vi "Na-DAS_7609.vi"(3 "Timeout (ms)":u32=10000, 5 "Input voltage range (V)":u8(ring)=1 items=["-5... +5 V", "-10... +10 V"]) -> (0 "DAQ Error":errorcluster, 1 "Overruns":u32, 2 "Config read-back ok":bool)   [LabVIEW 2014]
doc: "Use this plug-in with the Nathan 7609 data acquisition system"
uses:
  Globals/Meas_global.vi
  PWA/PWAtasksGLOBAL.vi
  Globals/Trav_pos_global.vi
  Globals/Extra_Commands_Global.vi
  Globals/Dynamic_call_global.ph.vi
panel:
  # "PN 25/11/2014, 19/12/2014"
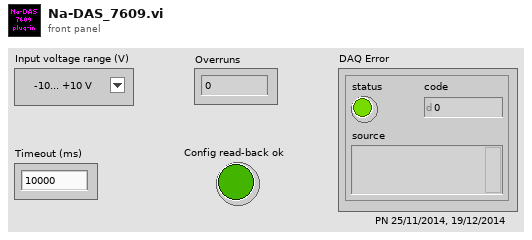
[diagram p1: front panel]
types:
  T1 = typedef "LDA_Setup.ctl" = cluster{"dimensions":enum16{"1D", "2D"}, "Analogue Freq Multiplier":dbl}
  T2 = typedef "Trigger_Mode.ctl" = enum16{"Free Running", "Start on Trigger", "Trigger Every Block", "Trigger Every Sample"}
  T3 = typedef "Traverse_cluster.ctl" = cluster{"Start X":dbl, "Start Y":dbl, "Start Z":dbl, "End X":dbl, "End Y":dbl, "End Z":dbl, "No. of pts.":i32, "Spacing":T4, "Filename":path, "Tunnel Speed":dbl, "Averaging time (min)":dbl, "Extra Commands":string, "Specific Arguments":string, "Emission Rate (l/min)":dbl, "Trace Gas Concentration (%)":dbl, "Density Ratio":string, "Comments":string, "Row No":i32, "Row Type Selector":T5, "Completion time":string, "Row Duration (mins)":dbl, "No. of Valid pts.":i32, "Meas Setup File":string}
  T4 = typedef "Spacing.ctl" = enum16{"Linear", "Log", "Gauss", "Specified", "N/A"}
  T5 = typedef "Multi_run_mode.ctl" = enum16{"Move Traverse Only", "Set Tunnel Speed Only", "Set Source Only", "Set Measurement Conditions", "Single Measurement", "Vertical Profile", "Lateral Profile", "Longitudinal Profile", "Explore Volume", "Multi-Axis Profile", "Auto Calibrate", "Meas Fast FID Bkgnd", "Check Beam Power", "Scanning Valve Measurement", "Run VI Named:", "Set ADAM Ch", "Wait (minutes)", "Send Message", "Synchronize With:", "Fall Back to this Row", "Turn Off Row Repeating", "Blank Row", "Traverse 3D Volume"}
  T6 = typedef "Ch_and_Spans.ctl" = cluster{"high limit (10V)":sgl, "low limit (-10V)":sgl, "Ch No":i16, "Var name":string, "Use Latest Calib":bool}
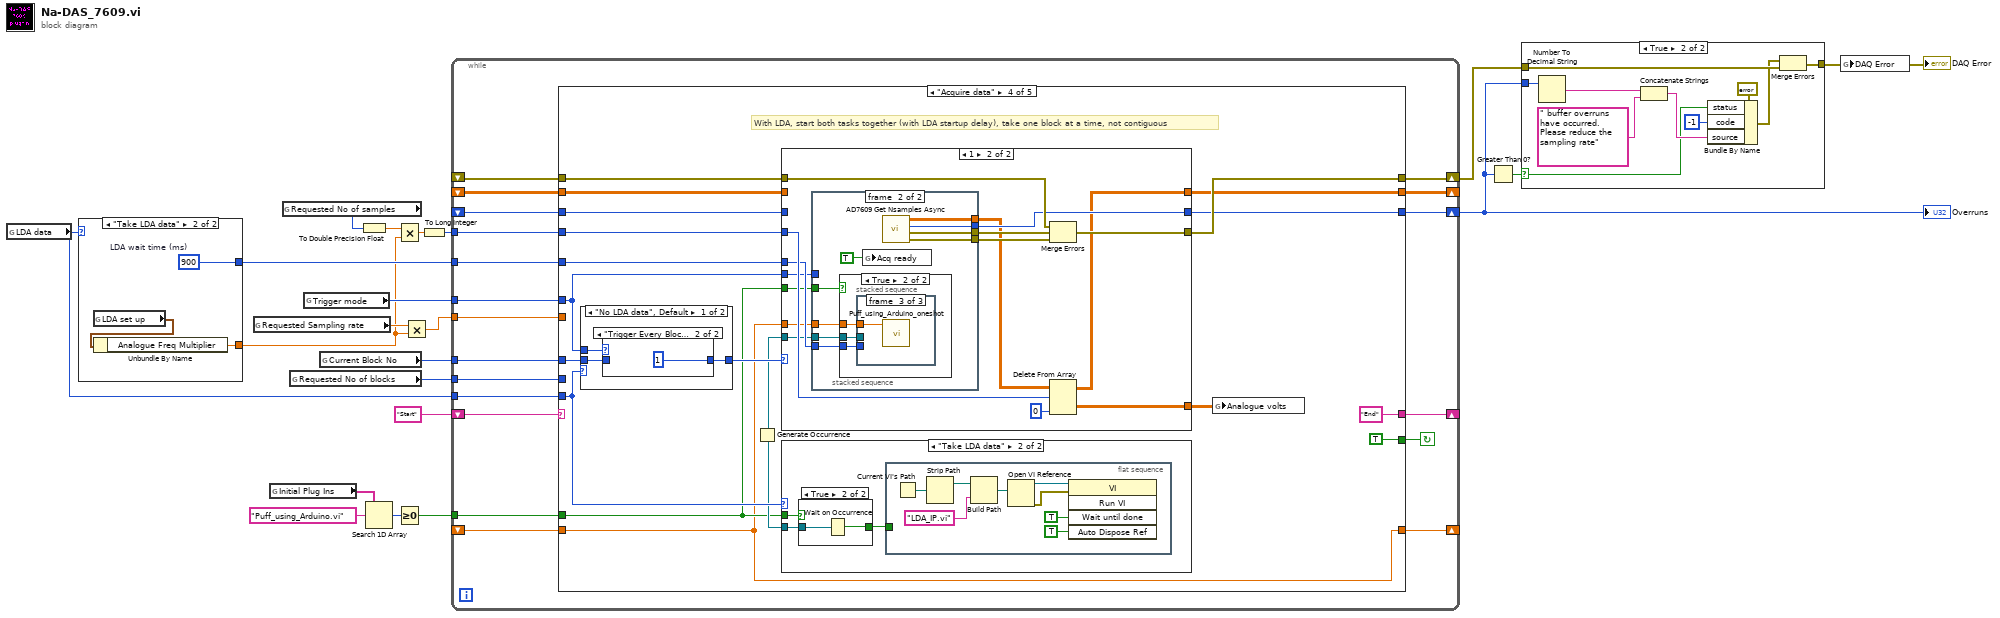
[diagram p0: block diagram]
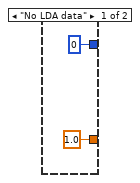
[diagram p3: hidden frame]
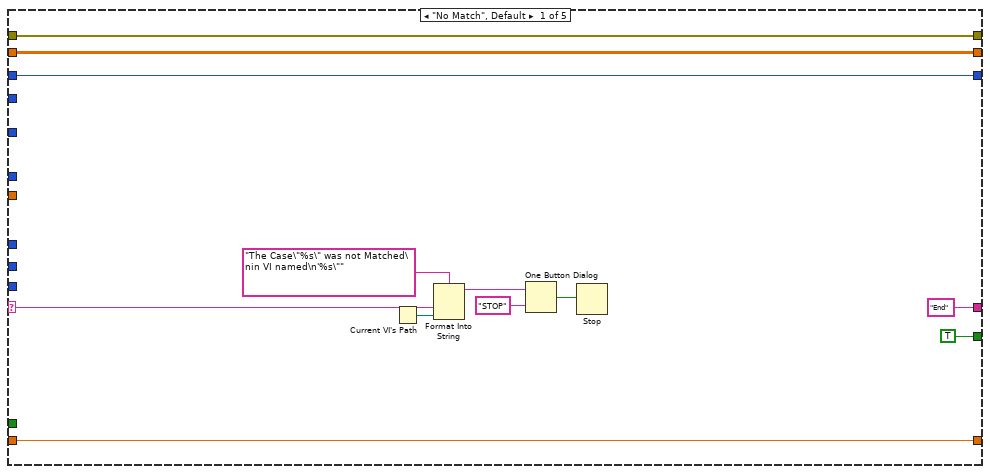
[diagram p4: hidden frame]
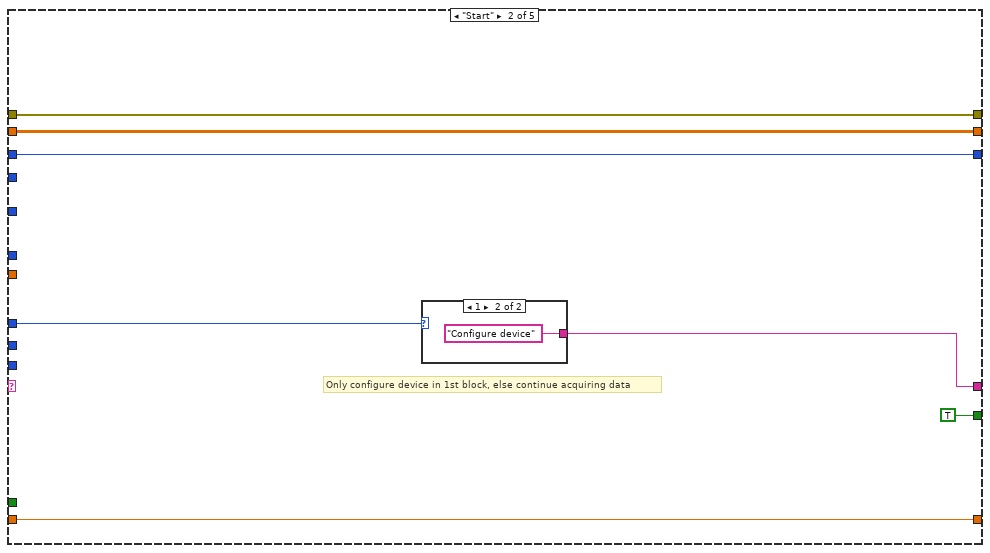
[diagram p5: hidden frame]
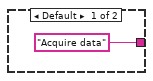
[diagram p6: hidden frame]
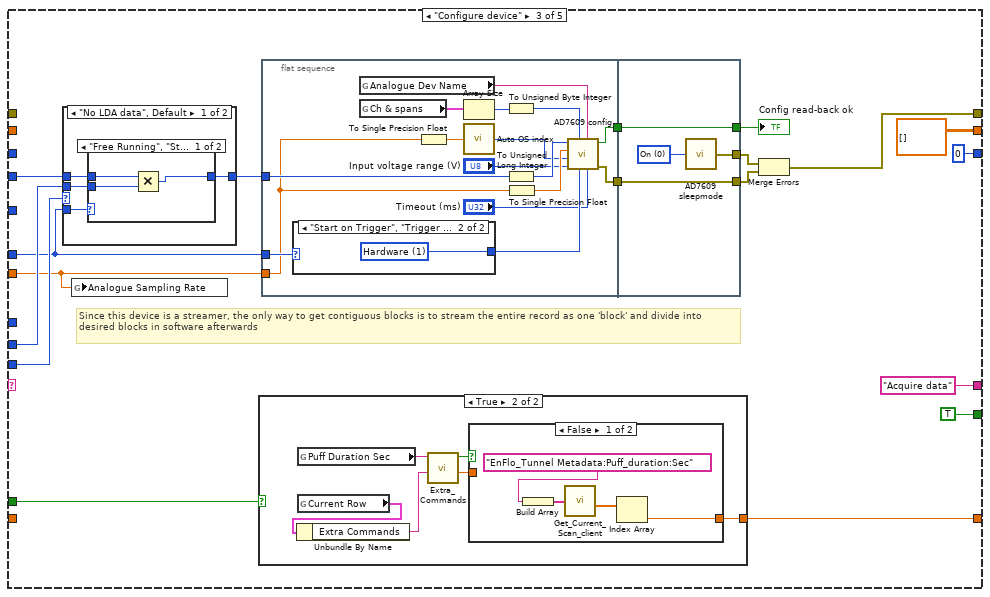
[diagram p7: hidden frame]
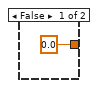
[diagram p8: hidden frame]
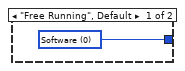
[diagram p12: hidden frame]
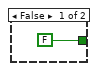
[diagram p14: hidden frame]
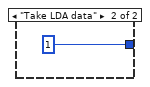
[diagram p16: hidden frame]
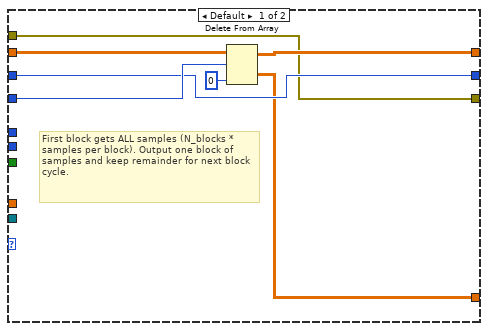
[diagram p17: hidden frame]
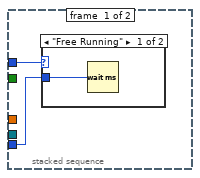
[diagram p18: hidden frame]
diagram:
  n1 = global read "Meas_global.vi" "LDA data"() -> (w16:enum16{"No LDA data", "Take LDA data"})
  n2 = case shown="\"Take LDA data\"" w16 {
    tunnel: [1.0 ("Analogue Freq Multiplier") w25] -> w5
    tunnel: [u32 0 ("LDA wait time (ms)") w24] -> w11
    frame "No LDA data" {
    }
    frame "Take LDA data" {
      w24 = u32 900  # LDA wait time (ms)
      n3 = global read "Meas_global.vi" "LDA set up"() -> (w26:T1)
      n4 = Unbundle By Name(w26) -> ("Analogue Freq Multiplier"=w25:dbl)
    }
  }
  n5 = global read "Meas_global.vi" "Requested Sampling rate"() -> (w17:dbl)
  n6 = global read "Dynamic_call_global.ph.vi" "Initial Plug Ins"() -> (w13:string[])
  n7 = global read "Meas_global.vi" "Requested No of samples"() -> (w6:i32)
  n8 = global read "Meas_global.vi" "Requested No of blocks"() -> (w1:i32)
  n9 = global read "Meas_global.vi" "Trigger mode"() -> (w20:T2)
  n10 = global read "Meas_global.vi" "Current Block No"() -> (w19:i32)
  n11 = To Double Precision Float(number=w6) -> (double precision float=w4:dbl)
  n12 = Search 1D Array(1D array=w13, element="Puff_using_Arduino.vi") -> (index of element=w15:i32)  [unwired: 1 in]
  n13 = Multiply(x=w4, y=w5) -> (x*y=w3:dbl)
  n14 = Greater Or Equal To 0?(x=w15) -> (x >= 0?=w12:bool)
  n15 = Multiply(x=w17, y=w5) -> (x*y=w18:dbl)
  n16 = To Long Integer(number=w3) -> (32bit integer=w2:i32)
  n17 = while {
    shift-left: "Start" -> [w45]
    shift-right: [w31] -> _
    tunnel: w18 -> [w44]
    tunnel: w2 -> [w43]
    tunnel: w19 -> [w42]
    tunnel: w20 -> [w40]
    tunnel: w16 -> [w39]
    tunnel: w1 -> [w38]
    shift-right: [w36] -> w10
    shift-left: _ -> [w37]
    shift-right: [w35] -> _
    shift-left: _ -> [w34]
    shift-right: [w33] -> w8
    shift-left: _ -> [w32]
    tunnel: w11 -> [w30]
    tunnel: w12 -> [w29]
    shift-right: [w28] -> _
    shift-left: _ -> [w27]
    stop <- w41 continue-if-true
    n18 = case shown="\"Acquire data\"" w45 {
      selector: w45 -> [w50 _ _ _ _]
      tunnel: ["End" w61 "Acquire data" ("f") "End" "End" ("f")] -> w31
      tunnel: w44 -> [_ _ w70 _ _]
      tunnel: w43 -> [_ _ w83 w139 _]
      tunnel: w42 -> [_ w62 _ w134 w212]
      tunnel: [TRUE TRUE TRUE TRUE FALSE] -> w41
      tunnel: w40 -> [_ _ w69 w128 _]
      tunnel: w39 -> [_ _ w81 w132 _]
      tunnel: w38 -> [_ _ w80 _ w213]
      tunnel: w37 -> [w49 w63 _ w143 w210]
      tunnel: [w49 w63 w82 w142 w209] -> w36
      tunnel: [w48 w60 dbl[][] [] ("Channel volts") w137 w208] -> w35
      tunnel: w34 -> [w48 w60 _ w138 w208]
      tunnel: [w47 w59 u32 0 ("Overruns") w141 w207] -> w33
      tunnel: w32 -> [w47 w59 _ w140 w207]
      tunnel: w30 -> [_ _ _ w133 _]
      tunnel: w29 -> [_ _ w68 w130 _]
      tunnel: [w46 w58 w67 w129 w206] -> w28
      tunnel: w27 -> [w46 w58 _ w129 w206]
      frame "No Match", Default {
        n19 = Current VI's Path() -> (path=w53:path)
        n20 = Format Into String(format string="The Case\"%s\" was not Matched\nin VI named\n'%s\"" ("Format String"), w50, w53) -> (resulting string=w56:string)  [unwired: 2 in, 1 out]
        n21 = One Button Dialog(message=w56, button name ("OK")="STOP") -> (true=w54:bool)
        n22 = Stop(stop? (T)=w54) -> ()
      }
      frame "Start" {
        # "Only configure device in 1st block, else continue acquiring data"
        n23 = case shown="1" w62 {
          tunnel: ["Acquire data" ("f") "Configure device" ("f")] -> w61
          frame Default {
          }
          frame 1 {
          }
        }
      }
      frame "Configure device" {
        # "Since this device is a streamer, the only way to get contiguous blocks is to stream the entire record as one 'block' and divide into desired blocks in software afterwards"
        n24 = case shown="\"No LDA data\", Default" w81 {
          tunnel: [w98 w105] -> w73
          tunnel: w83 -> [w100 w105]
          tunnel: w80 -> [w99 _]
          tunnel: w69 -> [w97 _]
          frame "No LDA data", Default {
            n25 = case shown="\"Free Running\", \"Start on Trigger\", Default" w97 {
              tunnel: w100 -> [w103 w104]
              tunnel: w99 -> [w102 _]
              tunnel: [w101 w104] -> w98
              frame "Free Running", "Start on Trigger", Default {
                n26 = Multiply(x=w103, y=w102) -> (x*y=w101:i32)
              }
              frame "Trigger Every Block" {
              }
            }
          }
          frame "Take LDA data" {
          }
        }
        n27 = global write "Meas_global.vi" "Analogue Sampling Rate"(w70) -> ()
        n28 = case shown="True" w68 {
          tunnel: [0.0 w91] -> w67
          frame False {
          }
          frame True {
            n29 = global read "Extra_Commands_Global.vi" "Puff Duration Sec"() -> (w88:string)
            n30 = global read "Trav_pos_global.vi" "Current Row"() -> (w90:T3)
            n31 = Unbundle By Name(w90) -> ("Extra Commands"=w89:string)
            n32 = call "Extra_Commands.vi"("String to Search"=w89, "Command"=w88) -> ("Numeric Value"=w86:dbl, "Command Found"=w87:bool)  [unwired: 2 in, 2 out]
            n33 = case shown="False" w87 {
              tunnel: [w92 w96] -> w91
              tunnel: w86 -> [_ w96]
              frame False {
                n34 = Build Array("EnFlo_Tunnel Metadata:Puff_duration:Sec") -> (w94:string[])
                n35 = call "Get_Current_Scan_client.vi"("ADAM Ch Names"=w94) -> ("Numerical Values"=w95:dbl[])  [unwired: 1 in, 2 out]
                n36 = Index Array(array=w95) -> (element=w92:dbl)  [unwired: 1 in]
              }
              frame True {
              }
            }
          }
        }
        n37 = flat-sequence {
          tunnel: w73 -> [w121]
          tunnel: w70 -> [w108]
          tunnel: w69 -> [w120]
          tunnel: [w114] -> w79
          tunnel: [w113] -> w78
          tunnel: [w126] -> w75
          tunnel: w79 -> [w126]
          tunnel: [w125] -> w77
          tunnel: w78 -> [w125]
          tunnel: [w124] -> w76
          frame #0 {
            n38 = case shown="\"Start on Trigger\", \"Trigger Every Block\"" w120 {
              tunnel: [w122 w123] -> w116
              frame "Free Running", Default {
                w122 = u8 0 items=["Software", "Hardware"] ("Triggering mode")
              }
              frame "Start on Trigger", "Trigger Every Block" {
                w123 = u8 1 items=["Software", "Hardware"] ("Triggering mode")
              }
            }
            n39 = global read "PWAtasksGLOBAL.vi" "Analogue Dev Name"() -> (w119:string)
            n40 = global read "Meas_global.vi" "Ch & spans"() -> (w112:T6[])
            n41 = To Single Precision Float(number=w108) -> (single precision float=w106:sgl)
            n42 = Array Size(array=w112) -> (size(s)=w111:i32)
            n43 = call "Auto OS index.vi"("Sampling rate"=w106) -> ("OS index"=w107:u8)
            n44 = To Unsigned Byte Integer(number=w111) -> (unsigned 8bit integer=w115:u8)
            n45 = To Unsigned Long Integer(number=w121) -> (unsigned 32bit integer=w118:u32)
            n46 = To Single Precision Float(number=w108) -> (single precision float=w117:sgl)
            n47 = call "AD7609 config.vi"("Timeout (ms)"="Timeout (ms)", "Device serial port"=w119, "Triggering mode"=w116, "N channels to read"=w115, "Input voltage range (V)"="Input voltage range (V)", "Oversampling ratio"=w107, "Sampling rate (Hz)"=w117, "Number of samples"=w118) -> ("Config error out"=w113:errorcluster, "Config read-back ok"=w114:bool)  [unwired: 2 in]
          }
          frame #1 {
            w127 = u8 0 items=["On", "Standby", "Shutdown"] ("Sleep state")
            n48 = call "AD7609 sleepmode.vi"("Sleep state"=w127) -> ("Sleep error out"=w124:errorcluster)
          }
        }
        n49 = Merge Errors(w76, w77) -> (w82:errorcluster)
        "Config read-back ok" <- w75
      }
      frame "Acquire data" {
        # "With LDA, start both tasks together (with LDA startup delay), take one block at a time, not contiguous"
        n50 = case shown="\"No LDA data\", Default" w132 {
          tunnel: w134 -> [w161 _]
          tunnel: w128 -> [w162 _]
          tunnel: [w160 1 ("Current Block No")] -> w135
          frame "No LDA data", Default {
            n51 = case shown="\"Trigger Every Block\"" w162 {
              tunnel: [w163 1 ("Current Block No")] -> w160
              tunnel: w161 -> [w163 _]
              frame "Free Running", "Start on Trigger", Default {
              }
              frame "Trigger Every Block" {
              }
            }
          }
          frame "Take LDA data" {
          }
        }
        n52 = Generate Occurrence() -> (w131:refnum<k4>)
        n53 = case shown="1" w135 {
          tunnel: w143 -> [w167 w185]
          tunnel: [w167 w184] -> w142
          tunnel: [w168 w183] -> w141
          tunnel: [w170 w180] -> w137
          tunnel: w139 -> [w169 w181]
          tunnel: w138 -> [w171 _]
          tunnel: w140 -> [w168 _]
          tunnel: [w166 w178] -> w136
          tunnel: w133 -> [_ w177]
          tunnel: w131 -> [_ w176]
          tunnel: w130 -> [_ w175]
          tunnel: w129 -> [_ w174]
          tunnel: w128 -> [_ w173]
          frame Default {
            # "First block gets ALL samples (N_blocks * samples per block). Output one block of samples and keep remainder for next block cycle."
            n54 = Delete From Array(array=w171, length=w169, index (col)=0 ("disabled index (col)")) -> (deleted portion=w166:dbl[][], array with subset deleted=w170:dbl[][])  [unwired: 1 in]
          }
          frame 1 {
            n55 = stacked-sequence {
              tunnel: [_ w198] -> w183
              tunnel: [_ w197] -> w182
              tunnel: [_ w196] -> w187
              tunnel: [_ w195] -> w186
              tunnel: w176 -> [_ w194]
              tunnel: w177 -> [w189 w193]
              tunnel: w175 -> [_ w192]
              tunnel: w174 -> [_ w191]
              tunnel: w173 -> [w188 _]
              frame #0 {
                n56 = case shown="\"Free Running\"" w188 {
                  tunnel: w189 -> [w190 _]
                  frame "Free Running" {
                    n57 = Wait (ms)(milliseconds to wait=w190) -> ()  [unwired: 1 out]
                  }
                  frame Default {
                  }
                }
              }
              frame #1 {
                n58 = case shown="True" w192 {
                  tunnel: w194 -> [_ w202]
                  tunnel: w191 -> [_ w201]
                  tunnel: w193 -> [_ w200]
                  frame False {
                  }
                  frame True {
                    n59 = stacked-sequence {
                      tunnel: w202 -> [w203 _ _]
                      tunnel: w201 -> [_ _ w205]
                      tunnel: w200 -> [_ w204 _]
                      frame #0 {
                        n60 = Set Occurrence(w203) -> ()
                      }
                      frame #1 {
                        n61 = Wait (ms)(milliseconds to wait=w204) -> ()  [unwired: 1 out]
                      }
                      frame #2 {
                        n62 = call "Puff_using_Arduino_oneshot.vi"("Puff_duration:Sec"=w205) -> ()  [unwired: 7 in]
                      }
                    }
                  }
                }
                n63 = global write "Meas_global.vi" "Acq ready"(TRUE ("Acq ready")) -> ()
                n64 = call "AD7609 Get Nsamples Async.vi"() -> ("Channel volts"=w197:dbl[][], "Overruns"=w198:u32, "Async error"=w195:errorcluster, "Overrun error out"=w196:errorcluster)  [unwired: 2 in]
              }
            }
            n65 = Merge Errors(w185, w186, w187) -> (w184:errorcluster)
            n66 = Delete From Array(array=w182, length=w181, index (col)=0 ("disabled index (col)")) -> (deleted portion=w178:dbl[][], array with subset deleted=w180:dbl[][])  [unwired: 1 in]
          }
        }
        n67 = case shown="\"Take LDA data\"" w132 {
          tunnel: w130 -> [_ w148]
          tunnel: w131 -> [_ w146]
          frame "No LDA data", Default {
          }
          frame "Take LDA data" {
            n68 = case shown="True" w148 {
              tunnel: w146 -> [_ w151]
              tunnel: [FALSE ("timed out") w150] -> w147
              frame False {
              }
              frame True {
                n69 = Wait on Occurrence(2:w151) -> (0:w150:bool)  [unwired: 2 in]
              }
            }
            n70 = flat-sequence {
              tunnel: w147 -> [_]
              frame #0 {
                n71 = Current VI's Path() -> (path=w153:path)
                n72 = Strip Path(path=w153) -> (stripped path=w152:path)  [unwired: 1 out]
                n73 = Build Path(base path=w152, name or relative path="LDA_IP.vi") -> (appended path=w154:path)
                n74 = Open VI Reference(vi path=w154) -> (vi reference=w157:refnum<vi>, error out=w158:errorcluster)  [unwired: 5 in]
                n75 = invoke class="VI" method="Run VI"(reference=w157, error in=w158, "Wait until done"=TRUE ("Wait Until Done"), "Auto Dispose Ref"=TRUE ("Wait until done")) -> ()  [unwired: 1 in, 5 out]
              }
            }
          }
        }
        n76 = global write "Meas_global.vi" "Analogue volts"(w136) -> ()
      }
      frame "End" {
        n77 = Equal?(x=w212, y=w213) -> (x = y?=w211:bool)
        n78 = case shown="True" w211 {
          tunnel: w210 -> [w217 w219]
          tunnel: [w217 w218] -> w209
          frame False {
          }
          frame True {
            w221 = u8 1 items=["On", "Standby", "Shutdown"] ("Sleep state")
            n79 = call "AD7609 sleepmode.vi"("Sleep state"=w221) -> ("Sleep error out"=w220:errorcluster)
            n80 = Merge Errors(w219, w220) -> (w218:errorcluster)
          }
        }
        n81 = global write "Meas_global.vi" "Acq ready"(FALSE ("Acq ready")) -> ()
      }
    }
  }
  "Overruns" <- w8
  n82 = Greater Than 0?(x=w8) -> (x > 0?=w7:bool)
  n83 = case shown="True" w7 {
    selector: w7 -> [_ w224]
    tunnel: w10 -> [w222 w231]
    tunnel: [w222 w232] -> w9
    tunnel: w8 -> [_ w230]
    frame False {
    }
    frame True {
      n84 = Number To Decimal String(number=w230) -> (decimal integer string=w228:string)  [unwired: 1 in]
      n85 = Concatenate Strings(w228, " buffer overruns have occurred. Please reduce the sampling rate") -> (w226:string)
      n86 = Bundle By Name(cluster=errorcluster {"status"=FALSE, "code"=0, "source"=""} ("error IO"), "status"=w224, "code"=-1, "source"=w226) -> (w223:errorcluster)
      n87 = Merge Errors(w223, w231) -> (w232:errorcluster)
    }
  }
  "DAQ Error" <- w9
  n88 = global write "Meas_global.vi" "DAQ Error"(w9) -> ()
